vi "exec ui.vi"(10 "EVENT":refnum<user-event>, 11 "DVR":refnum<data-value>) -> ()   [LabVIEW 2013, in "execution settings.lvclass"]
uses:
  execution settings.lvclass
  VI modification.lvclass
  execution settings.lvclass/execution settings.ctl
  Read allow debugging.vi
  Read auto error handling.vi
  Read Is Reentrant.vi
  Read Reentrancy Type.vi
panel:
  in  "Reentrancy Type":T1(ring)
  in  "Is Reentrant":bool
  in  "allow debugging":bool
  in  "auto error handling":bool
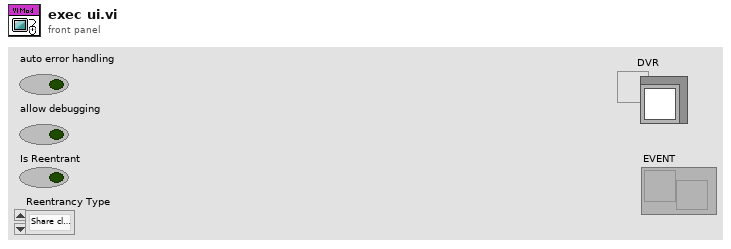
[diagram p1: front panel]
types:
  T1 = enum16{"Share clones between instances", "Preallocate clone for each instance"}
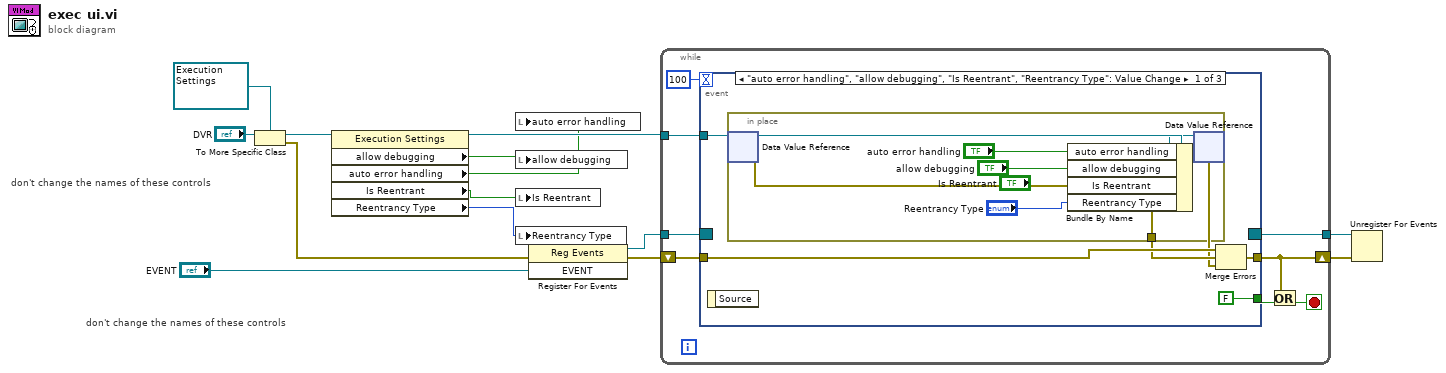
[diagram p0: block diagram]
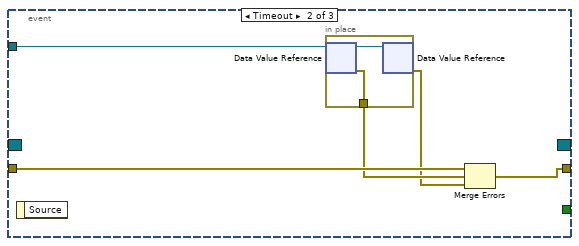
[diagram p2: hidden frame]
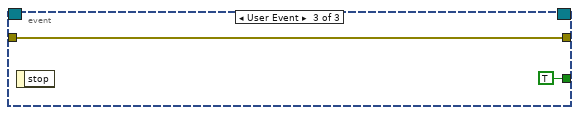
[diagram p3: hidden frame]
diagram:
  # "don't change the names of these controls"
  # "don't change the names of these controls"
  n1 = To More Specific Class(target class=refnum<data-value> refnum, reference="DVR") -> (specific class reference=w8:refnum<data-value>, error out=w6:errorcluster)  [unwired: 1 in]
  n2 = property class="Execution Settings"(reference=w8) -> (reference out=w5:refnum<data-value>, "allow debugging"=w4:bool, "auto error handling"=w3:bool, "Is Reentrant"=w2:bool, "Reentrancy Type"=w1:T1)  [unwired: 1 in, 1 out]
  n3 = local write "auto error handling"(w3) -> ()
  n4 = local write "allow debugging"(w4) -> ()
  n5 = local write "Is Reentrant"(w2) -> ()
  n6 = local write "Reentrancy Type"(w1) -> ()
  n7 = register-events(error in=w6, "EVENT") -> (reference out=w12:refnum<event-registration>, error out=w13:errorcluster)  [unwired: 1 in]
  n8 = while {
    shift-right: [w15] -> w11
    shift-left: w13 -> [w19]
    tunnel: w12 -> [w22]
    tunnel: [w21] -> w10
    tunnel: w5 -> [w18]
    stop <- w16 stop-if-true
    n9 = event shown="[0] \"auto error handling\", \"allow debugging\", \"Is Reentrant\", \"Reentrancy Type\": Value Change" {
      selector: w22 -> [_ _ _]
      dyn-events: [_ _ _] -> w21
      timeout: 100 -> [_ _ _]
      tunnel: [FALSE _ TRUE] -> w20
      tunnel: [w26 w38 w44] -> w15
      tunnel: w19 -> [w28 w39 w44]
      tunnel: w18 -> [w27 w40 _]
      event "auto error handling", "allow debugging", "Is Reentrant", "Reentrancy Type": Value Change {
        n10 = event-data() -> ()  [unwired: 1 in, 1 out]
        n11 = in-place {
          in-place-border: [w33] -> w24
          n12 = in-place-dvr #1(w27) -> (w35:refnum<class "execution settings.lvclass">, w33:errorcluster)
          n13 = Bundle By Name(cluster=w35, "auto error handling"="auto error handling", "allow debugging"="allow debugging", "Is Reentrant"="Is Reentrant", "Reentrancy Type"="Reentrancy Type") -> (w34:refnum<class "execution settings.lvclass">)
          n14 = in-place-dvr #1(w34) -> (w23:errorcluster)  [unwired: 1 out]
        }
        n15 = Merge Errors(w28, w24, w23) -> (w26:errorcluster)
      }
      event Timeout {
        n16 = event-data() -> ()  [unwired: 1 in, 1 out]
        n17 = in-place {
          in-place-border: [w41] -> w37
          n18 = in-place-dvr #2(w40) -> (w42:refnum<class "execution settings.lvclass">, w41:errorcluster)
          n19 = in-place-dvr #2(w42) -> (w36:errorcluster)  [unwired: 1 out]
        }
        n20 = Merge Errors(w39, w37, w36) -> (w38:errorcluster)
      }
      event User Event {
        n21 = event-data() -> ()  [unwired: 1 in, 1 out]
      }
    }
    n22 = Or(x=w15, y=w20) -> (x .or. y?=w16:bool)
  }
  n23 = Unregister For Events(event registration refnum=w10, error in=w11) -> ()  [unwired: 1 out]
